vi "FG_Press Map.vi"() -> (3 "Press Table":map{T1, string[]}(c390))   [LabVIEW 2024]
uses:
  Cluster_Start-End Keys.ctl
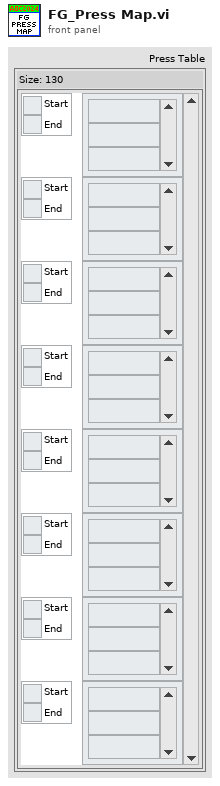
[diagram p1: front panel]
types:
  T1 = typedef "Cluster_Start-End Keys.ctl" = cluster{"Start":string, "End":string}
  T2 = typedef "Cluster_Row-Column.ctl" = cluster{"R":i32, "C":i32}
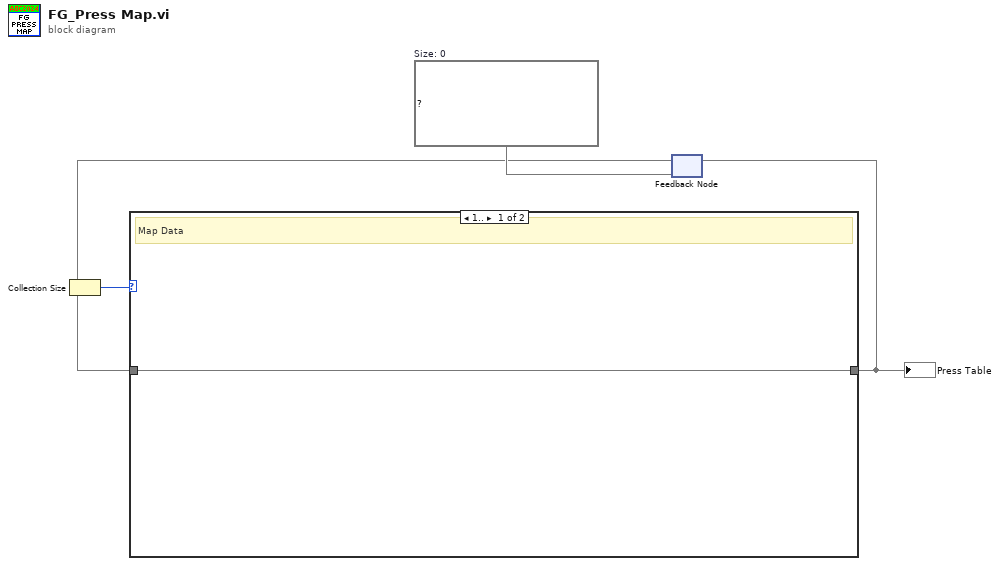
[diagram p0: block diagram]
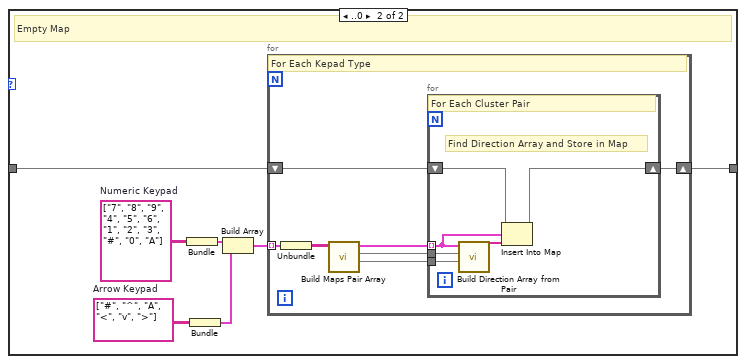
[diagram p2: hidden frame]
diagram:
  w2 = map{T1, string[]} {}  # Size: 0
  n1 = feedback #1(w2) -> (w1:map{T1, string[]})
  n2 = Collection Size(1:w1) -> (0:w3:i32)
  n3 = case shown="1.." w3 {
    tunnel: [w5 w7] -> w4
    tunnel: w1 -> [w5 w6]
    frame 1.. {
      # "Map Data"
    }
    frame ..0 {
      w10 = string[][] [["#", "^", "A"], ["<", "v", ">"]]  # Arrow Keypad
      w12 = string[][] [["7", "8", "9"], ["4", "5", "6"], ["1", "2", "3"], ["#", "0", "A"]]  # Numeric Keypad
      # "Empty Map"
      n4 = Bundle("Numeric Keypad"=w12) -> (w11:cluster{"Numeric Keypad":string[][]})  [unwired: 1 in]
      n5 = Bundle("Arrow Keypad"=w10) -> (w8:cluster{"Arrow Keypad":string[][]})  [unwired: 1 in]
      n6 = Build Array(w11, w8) -> (w9:cluster{"Arrow Keypad":string[][]}[])
      n7 = for {
        tunnel: w9 -> [w19] mode=indexing
        shift-right: [w16] -> w7
        shift-left: w6 -> [w18]
        # "For Each Kepad Type"
        n8 = Unbundle(w19) -> ("Arrow Keypad"=w17:string[][])
        n9 = call "Build Maps Pair Array.vi"("Keypad"=w17) -> ("Pos-Key Map Out"=w15:map{T2, string}, "Key-Pos Map Out"=w14:map{string, T2}, "Pair Array Out"=w13:T1[])  [unwired: 7 in, 1 out]
        n10 = for {
          tunnel: w13 -> [w21] mode=indexing
          tunnel: w14 -> [w25]
          tunnel: w15 -> [w20]
          shift-right: [w22] -> w16
          shift-left: w18 -> [w24]
          # "Find Direction Array and Store in Map"
          # "For Each Cluster Pair"
          n11 = call "Build Direction Array from Pair.vi"("Pos-Key Map Out"=w20, "Key-Pos Map Out"=w25, "output cluster"=w21) -> ("Direction Array"=w23:string[])  [unwired: 8 in]
          n12 = Insert Into Map(map in=w24, key=w21, value=w23) -> (map out=w22:map{T1, string[]})  [unwired: 2 out]
        }
      }
    }
  }
  "Press Table" <- w4
  n13 = feedback-in #1(w4) -> ()
